vi "CRYCalc mean and abs standard.vi"(6 "Work in":u16, 7 "Step Setup VI No":i32, 8 "Statistic Run Number":i32, 11 "Data in":T1 {"Z data" items=["dB", "Lin"]; "X data" items=["dB", "Lin"]; "Y data" items=["dB", "Lin"]; "Z dB ref" format="%.1f"; "Z axis" items=["Log", "Lin"]; "X dB ref" format="%.1f"; "X axis" items=["Log", "Lin"]; "Y axis" items=["Log", "Lin"]; "Y dB ref" format="%.1f"; "Curve"."z" format="%.2f"; "Curve"."y" format="%.2f"; "Curve"."x" format="%.2f"}) -> (0 "Out F":bool, 1 "Absolute StanDev Out":T1 {"Z data" items=["dB", "Lin"]; "X data" items=["dB", "Lin"]; "Y data" items=["dB", "Lin"]; "Z dB ref" format="%.1f"; "Z axis" items=["Log", "Lin"]; "X dB ref" format="%.1f"; "X axis" items=["Log", "Lin"]; "Y axis" items=["Log", "Lin"]; "Y dB ref" format="%.1f"; "Curve"."z" format="%.2f"; "Curve"."y" format="%.2f"; "Curve"."x" format="%.2f"}, 3 "Mean Out":T1 {"Z data" items=["dB", "Lin"]; "X data" items=["dB", "Lin"]; "Y data" items=["dB", "Lin"]; "Z dB ref" format="%.1f"; "Z axis" items=["Log", "Lin"]; "X dB ref" format="%.1f"; "X axis" items=["Log", "Lin"]; "Y axis" items=["Log", "Lin"]; "Y dB ref" format="%.1f"; "Curve"."z" format="%.2f"; "Curve"."y" format="%.2f"; "Curve"."x" format="%.2f"})   [LabVIEW 2013]
uses:
  Typedef Control/CRYData Cluster Array.ctl
  Typedef Control/CRYData Cluster.ctl
  <vilib>/Analysis/5stat.llb/RMS (DBL).vi
  CRYStatistics Global.vi
  <vilib>/Analysis/NI_AALBase.lvlib
  <vilib>/Analysis/NI_AALPro.lvlib
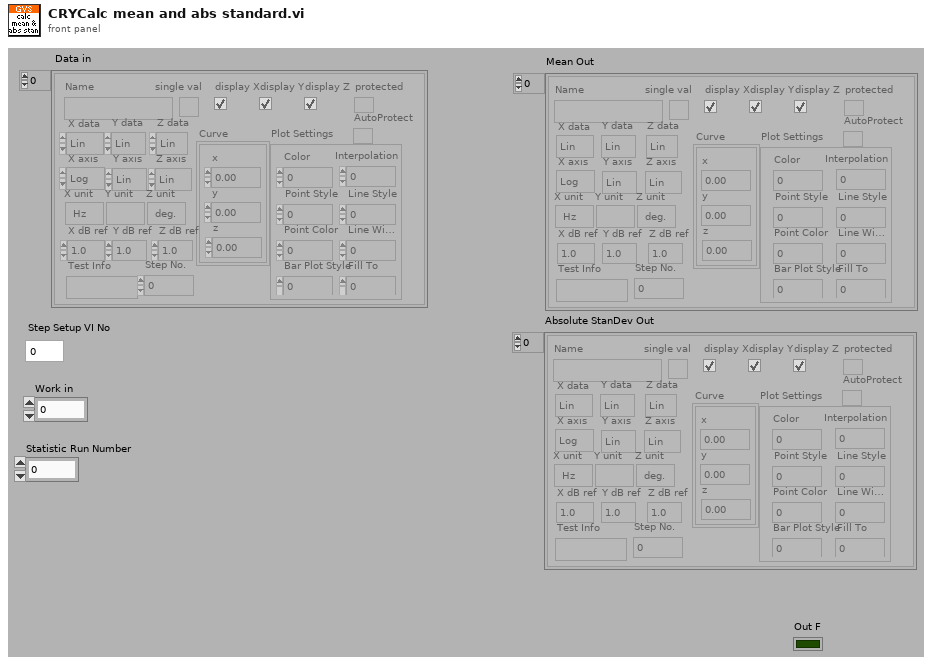
[diagram p1: front panel]
types:
  T1 = typedef "CRYData Cluster Array.ctl" = T2[]
  T2 = typedef "CRYData Cluster.ctl" = cluster{"Name":string, "Curve":cluster{"x":dbl, "y":dbl, "z":dbl}[], "X data":u16, "Y data":u16, "Z data":u16, "X axis":u16, "Y axis":u16, "Z axis":u16, "X unit":string, "Y unit":string, "Z unit":string, "X dB ref":dbl, "Y dB ref":dbl, "Z dB ref":dbl, "single val":bool, "protected":bool, "display X":bool, "display Y":bool, "display Z":bool, "Test Info":string, "Step No.":i32, "Plot Settings":cluster{"Color":u32, "Interpolation":u8, "Point Style":u8, "Line Style":u8, "Point Color":u32, "Line Width":u8, "Bar Plot Style":u8, "Fill To":i16}, "AutoProtect":bool}
  T3 = enum32{"English", "Chinese", "Korean", "Japanese", "Russian", "Chinese traditional"}
  T4 = cluster{"standard deviation":dbl, "standard deviation":dbl, "standard deviation":dbl}
  T5 = cluster{"mean":dbl, "rms value":dbl, "mean":dbl}[]
  T6 = cluster{"standard deviation":dbl, "standard deviation":dbl, "standard deviation":dbl}[]
  T7 = cluster{"x":dbl, "rms value":dbl, "rms value":dbl}
  T8 = cluster{"x":dbl, "standard deviation":dbl, "standard deviation":dbl}
  T9 = cluster{"x":dbl, "rms value":dbl, "rms value":dbl}[]
  T10 = cluster{"x":dbl, "standard deviation":dbl, "standard deviation":dbl}[]
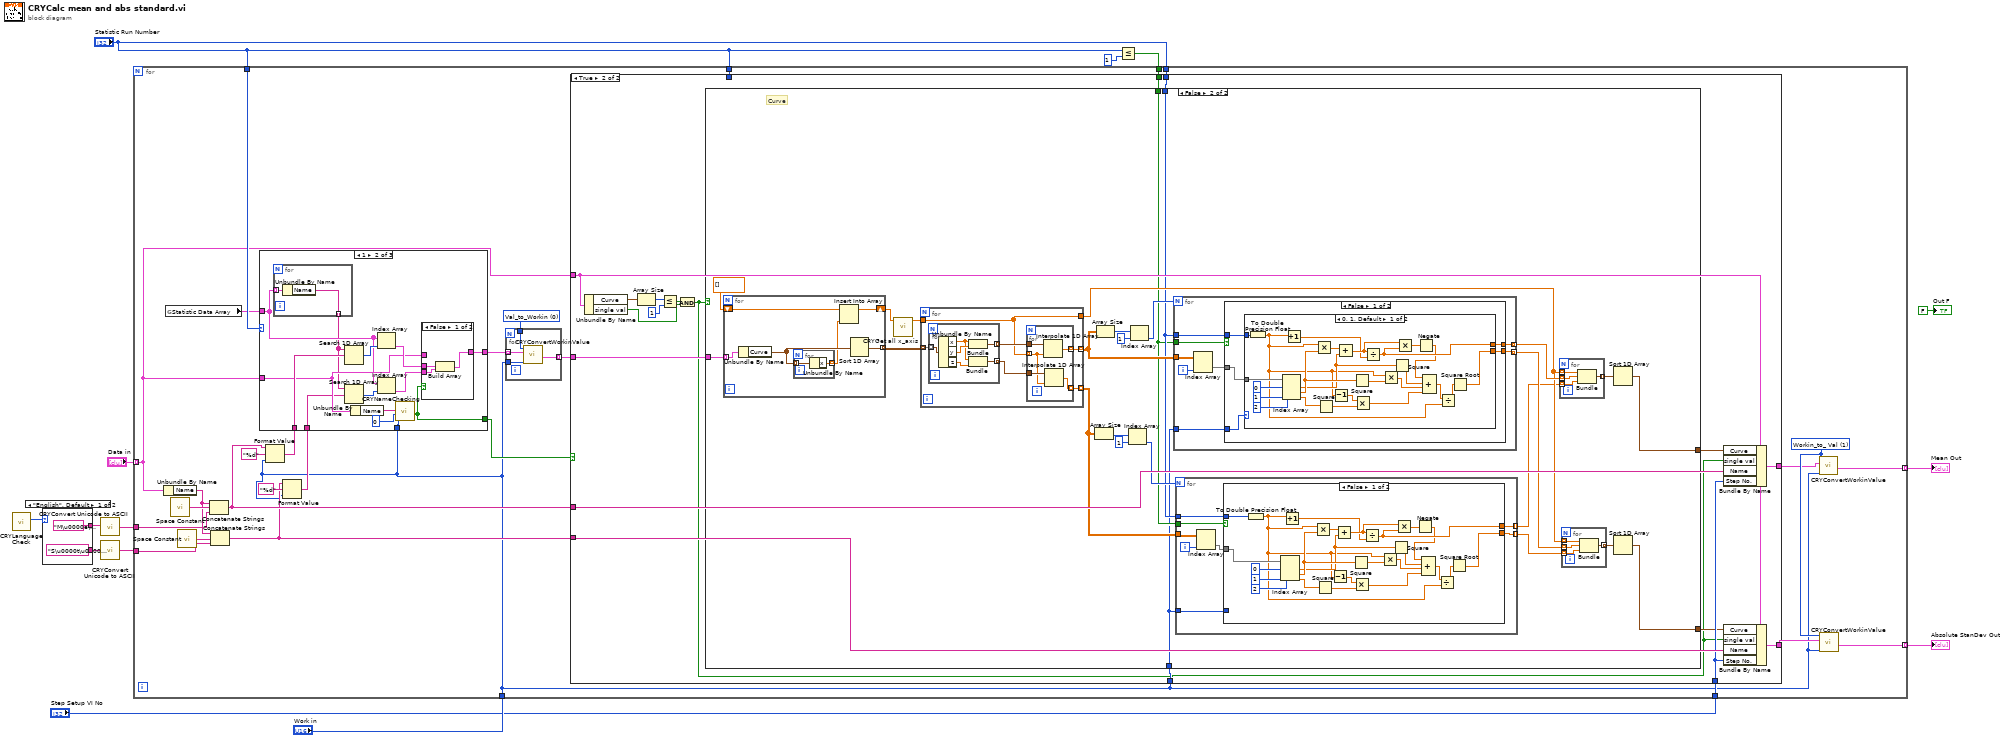
[diagram p0: block diagram]
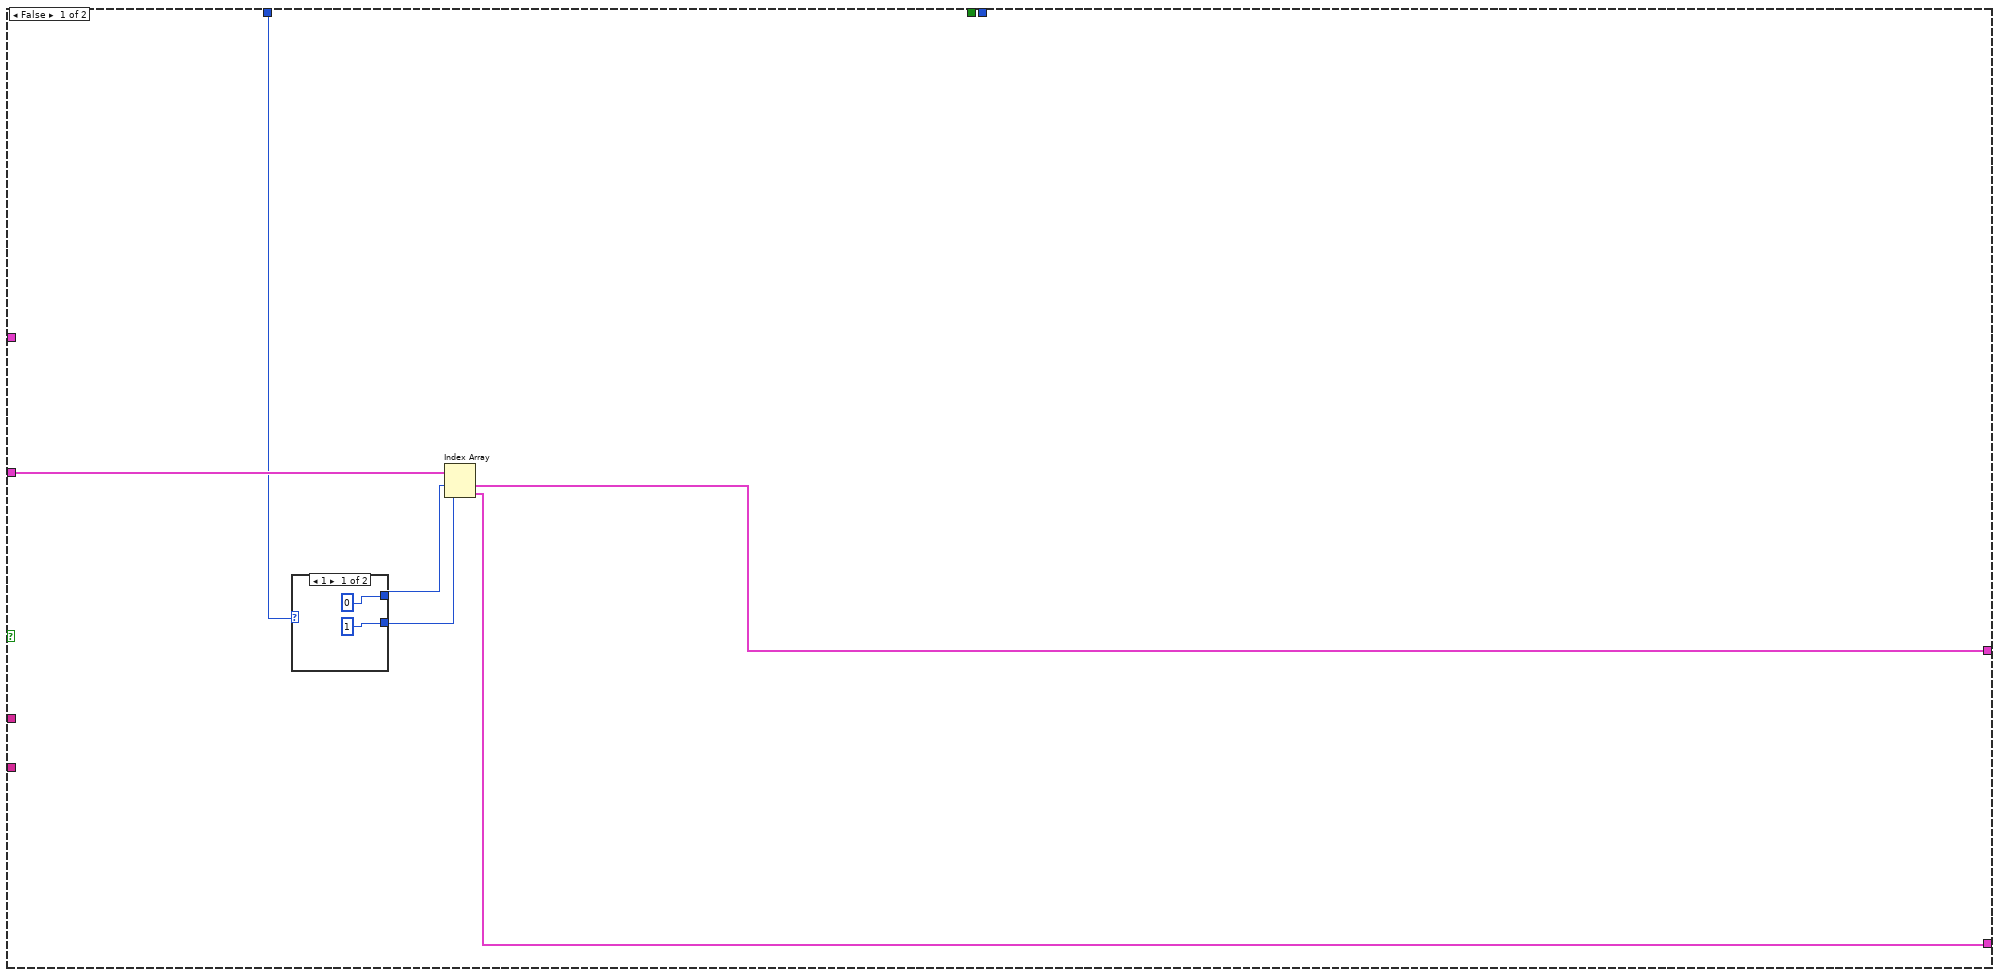
[diagram p2: hidden frame]
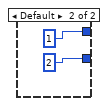
[diagram p3: hidden frame]
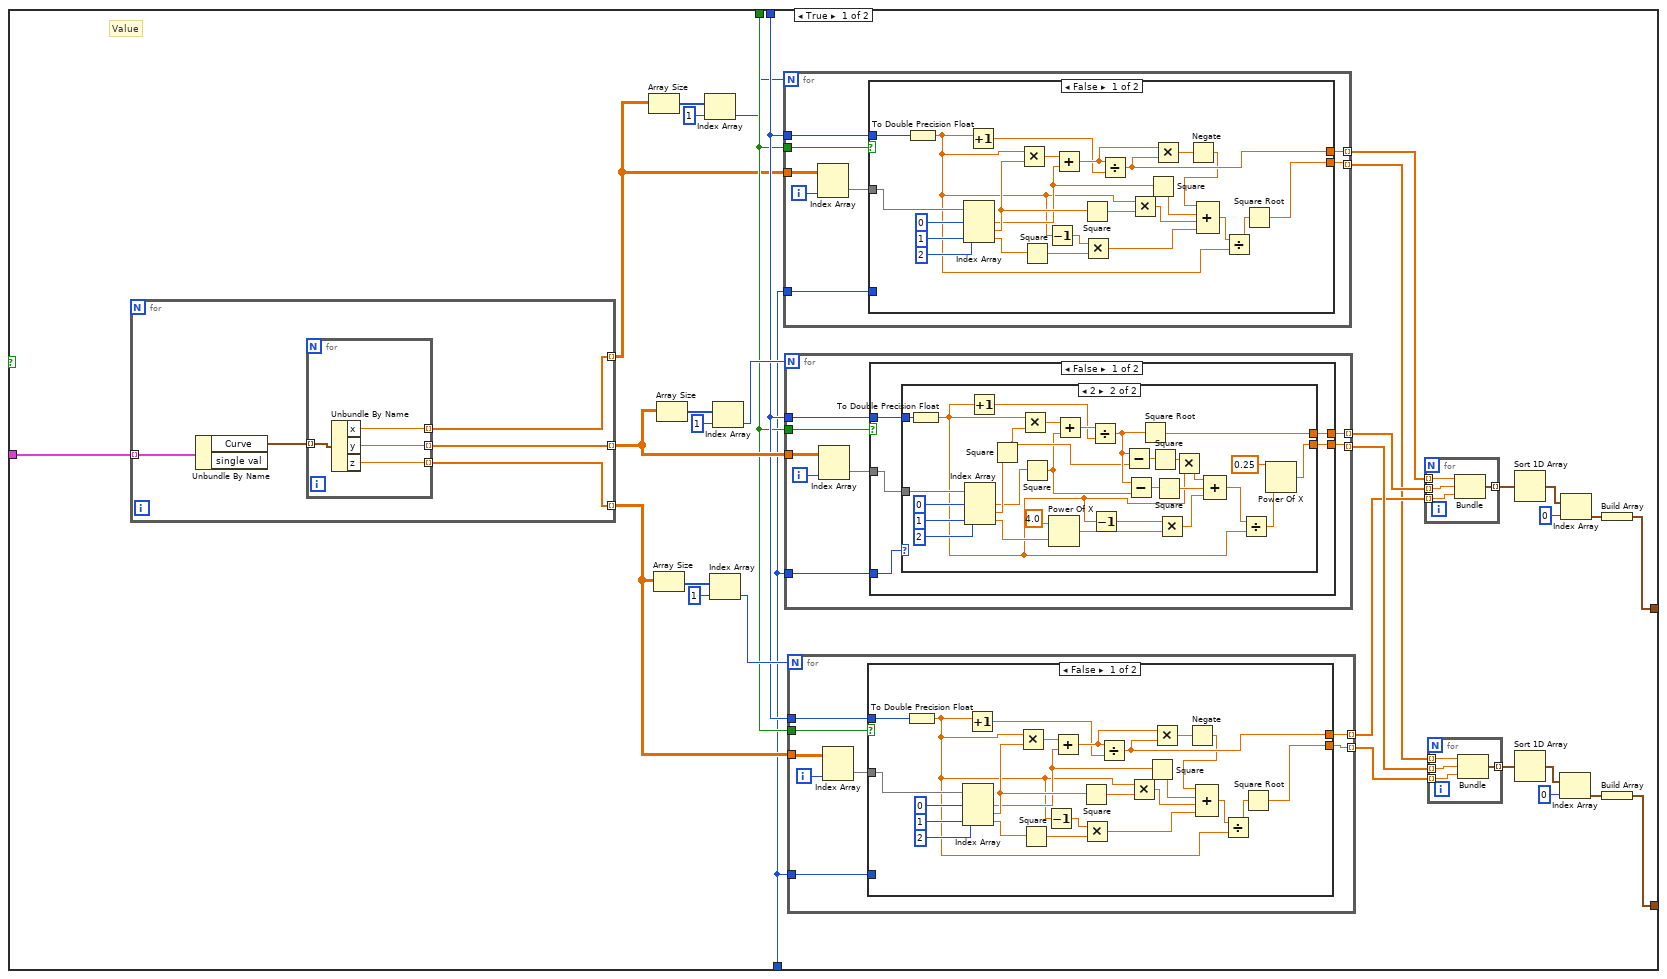
[diagram p4: hidden frame]
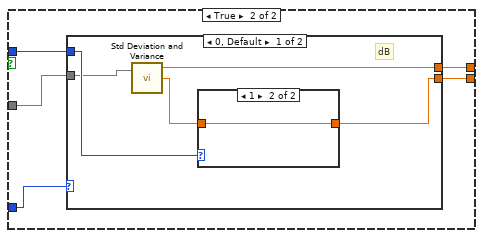
[diagram p5: hidden frame]
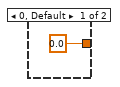
[diagram p6: hidden frame]
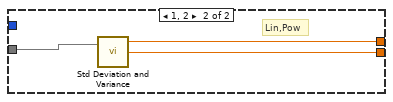
[diagram p7: hidden frame]
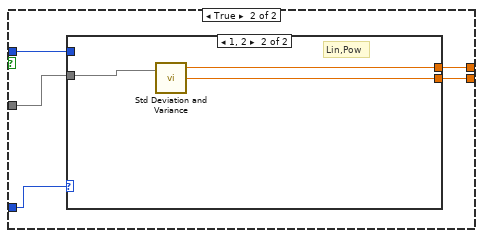
[diagram p8: hidden frame]
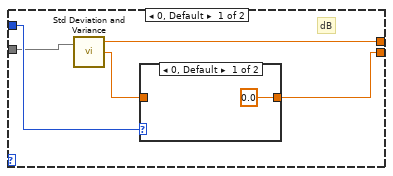
[diagram p9: hidden frame]
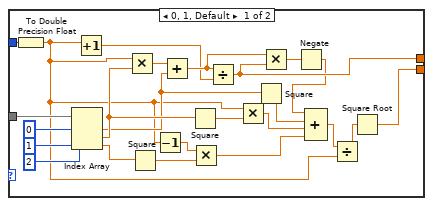
[diagram p11: hidden frame]
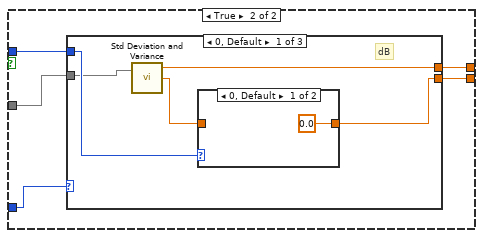
[diagram p12: hidden frame]
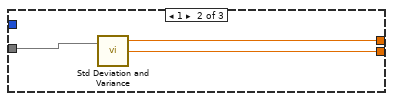
[diagram p14: hidden frame]
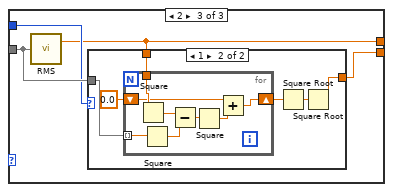
[diagram p15: hidden frame]
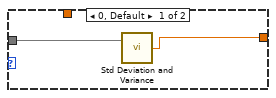
[diagram p16: hidden frame]
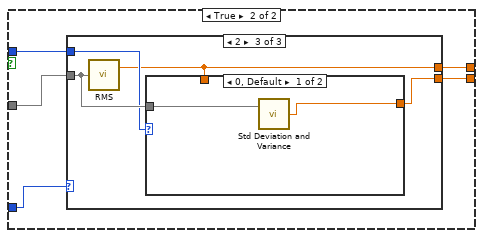
[diagram p17: hidden frame]
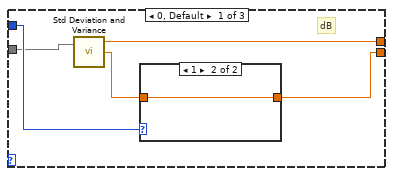
[diagram p18: hidden frame]
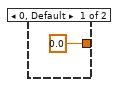
[diagram p19: hidden frame]
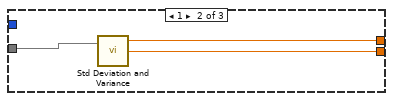
[diagram p20: hidden frame]
diagram:
  n1 = call "CRYLanguage Check.vi"() -> ("Language"=w9:T3)  [unwired: 10 in, 1 out]
  n2 = case shown="\"English\", Default" w9 {
    tunnel: ["M\u0000e\u0000a\u0000n\u0000" ("format string") "s^GW<P" ("format string")] -> w8
    tunnel: ["S\u0000t\u0000d\u0000 \u0000D\u0000e\u0000v\u0000" ("format string") "\u0007hÆQî]" ("format string")] -> w10
    frame "English", Default {
    }
    frame "Chinese" {
    }
  }
  n3 = call "CRYConvert Unicode to ASCII.vi"("Unicode"=w8) -> ("ASCII"=w7:string)  [unwired: 4 in]
  n4 = call "CRYConvert Unicode to ASCII.vi"("Unicode"=w10) -> ("ASCII"=w6:string)  [unwired: 4 in]
  n5 = Less Or Equal?(x="Statistic Run Number", y=1) -> (x <= y?=w4:bool)
  n6 = for {
    tunnel: "Data in" -> [w36] mode=indexing
    tunnel: [w27] -> w14 mode=indexing
    tunnel: w4 -> [w45]
    tunnel: "Statistic Run Number" -> [w46]
    tunnel: [w30] -> w13 mode=indexing
    tunnel: "Step Setup VI No" -> [w44]
    tunnel: "Statistic Run Number" -> [w43]
    tunnel: w7 -> [w38]
    tunnel: w6 -> [w37]
    tunnel: "Statistic Run Number" -> [w34]
    tunnel: "Work in" -> [w19]
    w31 = u16 1 items=["Val_to_Workin", "Workin_to_ Val"] ("Type")
    w33 = u16 0 items=["Val_to_Workin", "Workin_to_ Val"] ("Type")
    n7 = Unbundle By Name(w36) -> ("Name"=w40:string)
    n8 = global read "CRYStatistics Global.vi" "Statistic Data Array"() -> (w39:T1)
    n9 = call <vilib>:"Space Constant.vi"() -> ("String"=w42:string)
    n10 = call <vilib>:"Space Constant.vi"() -> ("String"=w41:string)
    n11 = Concatenate Strings(w40, w42, w38) -> (w24:string)
    n12 = Concatenate Strings(w40, w41, w37) -> (w21:string)
    n13 = Format Value(string ("")=w24, format string="%d", value (0)=w19) -> (output string=w23:string)
    n14 = Format Value(string ("")=w21, format string="%d", value (0)=w19) -> (output string=w20:string)
    n15 = case shown="1" w43 {
      tunnel: w36 -> [w550 w561 w578]
      tunnel: [w551 w564 w585] -> w29
      tunnel: w23 -> [_ w562 w586]
      tunnel: w20 -> [_ w556 w580]
      tunnel: w39 -> [_ w553 w581]
      tunnel: [TRUE ("Out Calcurated") w558 w579] -> w35
      tunnel: w19 -> [_ w554 w575]
      frame 0 {
        n16 = Build Array(w550, w550) -> (w551:T2[])
      }
      frame 1 {
        n17 = for {
          tunnel: w553 -> [w567] mode=indexing
          tunnel: [w566] -> w552 mode=indexing
          n18 = Unbundle By Name(w567) -> ("Name"=w566:string)
        }
        n19 = Search 1D Array(1D array=w552, element=w562) -> (index of element=w565:i32)  [unwired: 1 in]
        n20 = Search 1D Array(1D array=w552, element=w556) -> (index of element=w557:i32)  [unwired: 1 in]
        n21 = Unbundle By Name(w561) -> ("Name"=w560:string)
        n22 = Index Array(array=w553, index=w565) -> (element=w563:T2)
        n23 = Index Array(array=w553, index=w557) -> (element=w555:T2)
        n24 = call "CRYNameChecking.vi"("Curve Name"=w560, "Mode"=i8 0, "Work in"=w554) -> ("Out Calcurated"=w558:bool)  [unwired: 7 in]
        n25 = case shown="False" w558 {
          tunnel: [w568 w573] -> w564
          tunnel: w563 -> [w570 w572]
          tunnel: w561 -> [_ w571]
          tunnel: w555 -> [w569 _]
          frame False {
            n26 = Build Array(w570, w569) -> (w568:T2[])
          }
          frame True {
            n27 = Build Array(w571, w572) -> (w573:T2[])
          }
        }
      }
      frame Default {
        n28 = for {
          tunnel: w581 -> [w589] mode=indexing
          tunnel: [w588] -> w574 mode=indexing
          n29 = Unbundle By Name(w589) -> ("Name"=w588:string)
        }
        n30 = Unbundle By Name(w578) -> ("Name"=w577:string)
        n31 = Search 1D Array(1D array=w574, element=w586) -> (index of element=w587:i32)  [unwired: 1 in]
        n32 = Search 1D Array(1D array=w574, element=w580) -> (index of element=w583:i32)  [unwired: 1 in]
        n33 = Index Array(array=w581, index=w587) -> (element=w584:T2)
        n34 = Index Array(array=w581, index=w583) -> (element=w582:T2)
        n35 = call "CRYNameChecking.vi"("Curve Name"=w577, "Mode"=i8 0, "Work in"=w575) -> ("Out Calcurated"=w579:bool)  [unwired: 7 in]
        n36 = Build Array(w578, w584, w582) -> (w585:T2[])
      }
    }
    n37 = for {
      tunnel: w29 -> [w50] mode=indexing
      tunnel: [w49] -> w26 mode=indexing
      tunnel: w33 -> [w48]
      tunnel: w19 -> [w47]
      n38 = call "CRYConvertWorkinValue.vi"("Work in"=w47, "In"=w50, "Type"=w48) -> ("Out"=w49:T2)  [unwired: 8 in]
    }
    n39 = case shown="True" w35 {
      tunnel: [w56 w78] -> w28
      tunnel: w24 -> [_ w77]
      tunnel: w21 -> [_ w76]
      tunnel: [w55 w75] -> w32
      tunnel: w46 -> [_ w74]
      tunnel: w45 -> [_ w69]
      tunnel: w26 -> [w54 w73]
      tunnel: w44 -> [_ w72]
      tunnel: w36 -> [_ w62]
      tunnel: w34 -> [w53 _]
      tunnel: w19 -> [_ w68]
      frame False {
        n40 = case shown="1" w53 {
          tunnel: [0 1] -> w52
          tunnel: [1 2] -> w51
          frame 1 {
          }
          frame Default {
          }
        }
        n41 = Index Array(array=w54, index #1=w52, index #2=w51) -> (element #1=w56:T2, element #2=w55:T2)
      }
      frame True {
        n42 = Unbundle By Name(w62) -> ("Curve"=w67:cluster{"x":dbl, "y":dbl, "z":dbl}[], "single val"=w63:bool)
        n43 = Array Size(array=w67) -> (size(s)=w66:i32)
        n44 = Less Or Equal?(x=w66, y=1) -> (x <= y?=w64:bool)
        n45 = And(x=w64, y=w63) -> (x .and. y?=w61:bool)
        n46 = case shown="False" w61 {
          tunnel: w74 -> [w87 w331]
          tunnel: w73 -> [w92 w327]
          tunnel: [w95 w326] -> w71
          tunnel: [w93 w325] -> w70
          tunnel: w69 -> [w86 w324]
          tunnel: w68 -> [w85 w323]
          frame True {
            # "Value"
            n47 = for {
              tunnel: [w315] -> w110 mode=indexing
              tunnel: [w314] -> w99 mode=indexing
              tunnel: w92 -> [w318] mode=indexing
              tunnel: [w316] -> w81 mode=indexing
              n48 = Unbundle By Name(w318) -> ("Curve"=w317:cluster{"x":dbl, "y":dbl, "z":dbl}[])  [unwired: 1 out]
              n49 = for {
                tunnel: w317 -> [w322] mode=indexing
                tunnel: [w321] -> w316 mode=indexing
                tunnel: [w320] -> w315 mode=indexing
                tunnel: [w319] -> w314 mode=indexing
                n50 = Unbundle By Name(w322) -> ("x"=w321:dbl, "y"=w320:dbl, "z"=w319:dbl)
              }
            }
            n51 = Array Size(array=w81) -> (size(s)=w83:i32[])
            n52 = Array Size(array=w99) -> (size(s)=w103:i32[])
            n53 = Array Size(array=w110) -> (size(s)=w109:i32[])
            n54 = Index Array(array=w83, index=1) -> (element=w82:i32)
            n55 = Index Array(array=w103, index=1) -> (element=w100:i32)
            n56 = Index Array(array=w109, index=1) -> (element=w108:i32)
            n57 = for {
              N: w82 -> [_]
              tunnel: w81 -> [w118]
              tunnel: [w115] -> w79 mode=indexing
              tunnel: w86 -> [w114]
              tunnel: w87 -> [w113]
              tunnel: [w112] -> w80 mode=indexing
              tunnel: w85 -> [w111]
              i -> [w117]
              n58 = Index Array(array=w118, index (col)=w117) -> (element=w116:dbl[])  [unwired: 1 in]
              n59 = case shown="False" w114 {
                tunnel: w116 -> [w142 w147]
                tunnel: [w141 w146] -> w115
                tunnel: w113 -> [w139 w143]
                tunnel: [w140 w145] -> w112
                tunnel: w111 -> [_ w144]
                frame False {
                  n60 = To Double Precision Float(number=w139) -> (double precision float=w119:dbl)
                  n61 = Index Array(array=w142, index #1=0 ("index"), index #2=1 ("index"), index #3=2 ("index")) -> (element #1=w129:dbl, element #2=w131:dbl, element #3=w134:dbl)
                  n62 = Increment(x=w119) -> (x+1=w120:dbl)
                  n63 = Multiply(x=w119, y=w131) -> (x*y=w135:dbl)
                  n64 = Square(x=w134) -> (x^2=w132:dbl)
                  n65 = Decrement(x=w119) -> (x-1=w133:dbl)
                  n66 = Add(x=w135, y=w129) -> (x+y=w125:dbl)
                  n67 = Square(x=w131) -> (x^2=w130:dbl)
                  n68 = Multiply(x=w133, y=w132) -> (x*y=w126:dbl)
                  n69 = Divide(x=w125, y=w120) -> (x/y=w141:dbl)
                  n70 = Multiply(x=w119, y=w130) -> (x*y=w127:dbl)
                  n71 = Square(x=w129) -> (x^2=w128:dbl)
                  n72 = Multiply(x=w125, y=w141) -> (x*y=w124:dbl)
                  n73 = Negate(x=w124) -> (-x=w123:dbl)
                  n74 = Compound Arithmetic op=ADD(w123, w128, w127, w126) -> (w122:dbl)
                  n75 = Divide(x=w122, y=w119) -> (x/y=w121:dbl)
                  n76 = Square Root(x=w121) -> (sqrt(x)=w140:dbl)
                }
                frame True {
                  n77 = case shown="0, Default" w144 {
                    tunnel: w147 -> [w149 w157]
                    tunnel: [w152 w156] -> w146
                    tunnel: [w150 w155] -> w145
                    tunnel: w143 -> [w151 _]
                    frame 0, Default {
                      # "dB"
                      n78 = call <vilib>:"Std Deviation and Variance.vi"("X"=w149) -> ("mean"=w152:dbl, "standard deviation"=w148:dbl)  [unwired: 1 in, 1 out]
                      n79 = case shown="1" w151 {
                        tunnel: [0.0 w154] -> w150
                        tunnel: w148 -> [_ w154]
                        frame 0, Default {
                        }
                        frame 1 {
                        }
                      }
                    }
                    frame 1, 2 {
                      # "Lin,Pow"
                      n80 = call <vilib>:"Std Deviation and Variance.vi"("X"=w157) -> ("mean"=w156:dbl, "standard deviation"=w155:dbl)  [unwired: 1 in, 1 out]
                    }
                  }
                }
              }
            }
            n81 = for {
              N: w108 -> [_]
              tunnel: w110 -> [w220]
              tunnel: [w217] -> w106 mode=indexing
              tunnel: w86 -> [w216]
              tunnel: w87 -> [w215]
              tunnel: [w214] -> w101 mode=indexing
              tunnel: w85 -> [w213]
              i -> [w219]
              n82 = Index Array(array=w220, index (col)=w219) -> (element=w218:dbl[])  [unwired: 1 in]
              n83 = case shown="False" w216 {
                tunnel: w218 -> [w225 w283]
                tunnel: [w224 w282] -> w217
                tunnel: w215 -> [w222 w279]
                tunnel: [w223 w281] -> w214
                tunnel: w213 -> [w221 w280]
                frame False {
                  n84 = case shown="2" w221 {
                    tunnel: w225 -> [w249 w278]
                    tunnel: [w234 w269] -> w224
                    tunnel: [w230 w261] -> w223
                    tunnel: w222 -> [w228 w264]
                    frame 0, 1, Default {
                      n85 = To Double Precision Float(number=w228) -> (double precision float=w226:dbl)
                      n86 = Index Array(array=w249, index #1=0 ("index"), index #2=1 ("index"), index #3=2 ("index")) -> (element #1=w239:dbl, element #2=w241:dbl, element #3=w244:dbl)
                      n87 = Increment(x=w226) -> (x+1=w227:dbl)
                      n88 = Multiply(x=w226, y=w241) -> (x*y=w245:dbl)
                      n89 = Square(x=w244) -> (x^2=w242:dbl)
                      n90 = Decrement(x=w226) -> (x-1=w243:dbl)
                      n91 = Add(x=w245, y=w239) -> (x+y=w235:dbl)
                      n92 = Square(x=w241) -> (x^2=w240:dbl)
                      n93 = Multiply(x=w243, y=w242) -> (x*y=w236:dbl)
                      n94 = Divide(x=w235, y=w227) -> (x/y=w234:dbl)
                      n95 = Multiply(x=w226, y=w240) -> (x*y=w237:dbl)
                      n96 = Square(x=w239) -> (x^2=w238:dbl)
                      n97 = Multiply(x=w235, y=w234) -> (x*y=w233:dbl)
                      n98 = Negate(x=w233) -> (-x=w232:dbl)
                      n99 = Compound Arithmetic op=ADD(w232, w238, w237, w236) -> (w231:dbl)
                      n100 = Divide(x=w231, y=w226) -> (x/y=w229:dbl)
                      n101 = Square Root(x=w229) -> (sqrt(x)=w230:dbl)
                    }
                    frame 2 {
                      n102 = To Double Precision Float(number=w264) -> (double precision float=w251:dbl)
                      n103 = Index Array(array=w278, index #1=0 ("index"), index #2=1 ("index"), index #3=2 ("index")) -> (element #1=w272:dbl, element #2=w273:dbl, element #3=w268:dbl)
                      n104 = Increment(x=w251) -> (x+1=w254:dbl)
                      n105 = Square(x=w273) -> (x^2=w257:dbl)
                      n106 = Multiply(x=w251, y=w257) -> (x*y=w274:dbl)
                      n107 = Square(x=w272) -> (x^2=w256:dbl)
                      n108 = Power Of X(1:w268, 2:4.0 ("y")) -> (0:w266:dbl)
                      n109 = Add(x=w274, y=w256) -> (x+y=w271:dbl)
                      n110 = Divide(x=w271, y=w254) -> (x/y=w258:dbl)
                      n111 = Decrement(x=w251) -> (x-1=w250:dbl)
                      n112 = Subtract(x=w258, y=w257) -> (x-y=w259:dbl)
                      n113 = Subtract(x=w258, y=w256) -> (x-y=w253:dbl)
                      n114 = Square Root(x=w258) -> (sqrt(x)=w269:dbl)
                      n115 = Square(x=w259) -> (x^2=w260:dbl)
                      n116 = Square(x=w253) -> (x^2=w252:dbl)
                      n117 = Multiply(x=w250, y=w266) -> (x*y=w265:dbl)
                      n118 = Multiply(x=w260, y=w251) -> (x*y=w255:dbl)
                      n119 = Compound Arithmetic op=ADD(w255, w252, w265) -> (w270:dbl)
                      n120 = Divide(x=w270, y=w251) -> (x/y=w263:dbl)
                      n121 = Power Of X(1:w263, 2:0.25 ("y")) -> (0:w261:dbl)
                    }
                  }
                }
                frame True {
                  n122 = case shown="0, Default" w280 {
                    tunnel: w283 -> [w285 w293 w296]
                    tunnel: [w288 w292 w294] -> w282
                    tunnel: [w286 w291 w297] -> w281
                    tunnel: w279 -> [w287 _ w295]
                    frame 0, Default {
                      # "dB"
                      n123 = call <vilib>:"Std Deviation and Variance.vi"("X"=w285) -> ("mean"=w288:dbl, "standard deviation"=w284:dbl)  [unwired: 1 in, 1 out]
                      n124 = case shown="0, Default" w287 {
                        tunnel: [0.0 w290] -> w286
                        tunnel: w284 -> [_ w290]
                        frame 0, Default {
                        }
                        frame 1 {
                        }
                      }
                    }
                    frame 1 {
                      n125 = call <vilib>:"Std Deviation and Variance.vi"("X"=w293) -> ("mean"=w292:dbl, "standard deviation"=w291:dbl)  [unwired: 1 in, 1 out]
                    }
                    frame 2 {
                      n126 = call-poly <vilib>:"RMS.vi"("X"=w296) -> ("rms value"=w294:dbl)  [unwired: 1 out]
                      n127 = case shown="1" w295 {
                        tunnel: [w298 w300] -> w297
                        tunnel: w296 -> [w299 w304]
                        tunnel: w294 -> [_ w303]
                        frame 0, Default {
                          n128 = call <vilib>:"Std Deviation and Variance.vi"("X"=w299) -> ("standard deviation"=w298:dbl)  [unwired: 1 in, 2 out]
                        }
                        frame 1 {
                          n129 = for {
                            tunnel: w304 -> [w312] mode=indexing
                            tunnel: w303 -> [w313]
                            shift-right: [w308] -> w302
                            shift-left: 0.0 -> [w307]
                            n130 = Square(x=w313) -> (x^2=w311:dbl)
                            n131 = Square(x=w312) -> (x^2=w310:dbl)
                            n132 = Subtract(x=w311, y=w310) -> (x-y=w309:dbl)
                            n133 = Square(x=w309) -> (x^2=w306:dbl)
                            n134 = Add(x=w307, y=w306) -> (x+y=w308:dbl)
                          }
                          n135 = Square Root(x=w302) -> (sqrt(x)=w301:dbl)
                          n136 = Square Root(x=w301) -> (sqrt(x)=w300:dbl)
                        }
                      }
                    }
                  }
                }
              }
            }
            n137 = for {
              N: w100 -> [_]
              tunnel: w99 -> [w165]
              tunnel: [w160] -> w98 mode=indexing
              tunnel: w86 -> [w162]
              tunnel: w87 -> [w163]
              tunnel: [w159] -> w97 mode=indexing
              tunnel: w85 -> [w161]
              i -> [w164]
              n138 = Index Array(array=w165, index (col)=w164) -> (element=w158:dbl[])  [unwired: 1 in]
              n139 = case shown="False" w162 {
                tunnel: w158 -> [w189 w194]
                tunnel: [w188 w193] -> w160
                tunnel: w163 -> [w186 w190]
                tunnel: [w187 w192] -> w159
                tunnel: w161 -> [_ w191]
                frame False {
                  n140 = To Double Precision Float(number=w186) -> (double precision float=w166:dbl)
                  n141 = Index Array(array=w189, index #1=0 ("index"), index #2=1 ("index"), index #3=2 ("index")) -> (element #1=w176:dbl, element #2=w178:dbl, element #3=w181:dbl)
                  n142 = Increment(x=w166) -> (x+1=w167:dbl)
                  n143 = Multiply(x=w166, y=w178) -> (x*y=w182:dbl)
                  n144 = Square(x=w181) -> (x^2=w179:dbl)
                  n145 = Decrement(x=w166) -> (x-1=w180:dbl)
                  n146 = Add(x=w182, y=w176) -> (x+y=w172:dbl)
                  n147 = Square(x=w178) -> (x^2=w177:dbl)
                  n148 = Multiply(x=w180, y=w179) -> (x*y=w173:dbl)
                  n149 = Divide(x=w172, y=w167) -> (x/y=w188:dbl)
                  n150 = Multiply(x=w166, y=w177) -> (x*y=w174:dbl)
                  n151 = Square(x=w176) -> (x^2=w175:dbl)
                  n152 = Multiply(x=w172, y=w188) -> (x*y=w171:dbl)
                  n153 = Negate(x=w171) -> (-x=w170:dbl)
                  n154 = Compound Arithmetic op=ADD(w170, w175, w174, w173) -> (w169:dbl)
                  n155 = Divide(x=w169, y=w166) -> (x/y=w168:dbl)
                  n156 = Square Root(x=w168) -> (sqrt(x)=w187:dbl)
                }
                frame True {
                  n157 = case shown="1, 2" w191 {
                    tunnel: w194 -> [w196 w204]
                    tunnel: [w199 w203] -> w193
                    tunnel: [w197 w202] -> w192
                    tunnel: w190 -> [w198 _]
                    frame 0, Default {
                      # "dB"
                      n158 = call <vilib>:"Std Deviation and Variance.vi"("X"=w196) -> ("mean"=w199:dbl, "standard deviation"=w195:dbl)  [unwired: 1 in, 1 out]
                      n159 = case shown="0, Default" w198 {
                        tunnel: [0.0 w201] -> w197
                        tunnel: w195 -> [_ w201]
                        frame 0, Default {
                        }
                        frame 1 {
                        }
                      }
                    }
                    frame 1, 2 {
                      # "Lin,Pow"
                      n160 = call <vilib>:"Std Deviation and Variance.vi"("X"=w204) -> ("mean"=w203:dbl, "standard deviation"=w202:dbl)  [unwired: 1 in, 1 out]
                    }
                  }
                }
              }
            }
            n161 = for {
              tunnel: w106 -> [w211] mode=indexing
              tunnel: [w212] -> w105 mode=indexing
              tunnel: w79 -> [w210] mode=indexing
              tunnel: w98 -> [w209] mode=indexing
              n162 = Bundle("mean"=w210, "rms value"=w211, "mean"=w209) -> (w212:cluster{"mean":dbl, "rms value":dbl, "mean":dbl})  [unwired: 1 out]
            }
            n163 = for {
              tunnel: w101 -> [w207] mode=indexing
              tunnel: [w208] -> w102 mode=indexing
              tunnel: w80 -> [w206] mode=indexing
              tunnel: w97 -> [w205] mode=indexing
              n164 = Bundle("standard deviation"=w206, "standard deviation"=w207, "standard deviation"=w205) -> (w208:T4)  [unwired: 1 out]
            }
            n165 = Sort 1D Array(array=w105) -> (sorted array=w96:T5)
            n166 = Sort 1D Array(array=w102) -> (sorted array=w94:T6)
            n167 = Index Array(array=w94, index=0) -> (element=w88:T4)
            n168 = Index Array(array=w96, index=0) -> (element=w90:cluster{"mean":dbl, "rms value":dbl, "mean":dbl})
            n169 = Build Array(w90) -> (w95:T5)
            n170 = Build Array(w88) -> (w93:T6)
          }
          frame False {
            # "Curve"
            n171 = for {
              tunnel: [w524] -> w345 mode=indexing
              tunnel: w327 -> [w525] mode=indexing
              shift-right: [w527] -> w338
              shift-left: dbl[] [] ("x_Array") -> [w526]
              n172 = Unbundle By Name(w525) -> ("Curve"=w529:cluster{"x":dbl, "y":dbl, "z":dbl}[])
              n173 = for {
                tunnel: w529 -> [w530] mode=indexing
                tunnel: [w531] -> w528 mode=indexing
                n174 = Unbundle By Name(w530) -> ("x"=w531:dbl)
              }
              n175 = Insert Into Array(array=w526, new element=w528) -> (w527:dbl[])  [unwired: 1 in]
              n176 = Sort 1D Array(array=w529) -> (sorted array=w524:cluster{"x":dbl, "y":dbl, "z":dbl}[])
            }
            n177 = call "CRYGet all x_axis.vi"("x_Array in"=w338) -> ("X_axis out"=w344:dbl[])  [unwired: 1 in, 9 out]
            n178 = for {
              tunnel: w345 -> [w533] mode=indexing
              tunnel: [w537] -> w347 mode=indexing
              tunnel: w344 -> [w532]
              tunnel: [w532] -> w334
              tunnel: [w534] -> w330 mode=indexing
              n179 = for {
                tunnel: [w542] -> w536 mode=indexing
                tunnel: w533 -> [w541] mode=indexing
                tunnel: [w538] -> w535 mode=indexing
                n180 = Unbundle By Name(w541) -> ("x"=w539:dbl, "y"=w543:dbl, "z"=w540:dbl)
                n181 = Bundle("x"=w539, "z"=w540) -> (w538:cluster{"x":dbl, "z":dbl})  [unwired: 1 out]
                n182 = Bundle("x"=w539, "y"=w543) -> (w542:cluster{"x":dbl, "y":dbl})  [unwired: 1 out]
              }
              n183 = for {
                tunnel: [w548] -> w537 mode=indexing
                tunnel: w536 -> [w547]
                tunnel: w532 -> [w545] mode=indexing
                tunnel: w535 -> [w546]
                tunnel: [w544] -> w534 mode=indexing
                n184 = Interpolate 1D Array(1:w545, 2:w547) -> (0:w548:dbl)
                n185 = Interpolate 1D Array(1:w545, 2:w546) -> (0:w544:dbl)
              }
            }
            n186 = Array Size(array=w330) -> (size(s)=w336:i32[])
            n187 = Array Size(array=w347) -> (size(s)=w343:i32[])
            n188 = Index Array(array=w336, index=1) -> (element=w332:i32)
            n189 = Index Array(array=w343, index=1) -> (element=w342:i32)
            n190 = for {
              N: w342 -> [_]
              tunnel: w347 -> [w430]
              tunnel: [w427] -> w340 mode=indexing
              tunnel: w324 -> [w426]
              tunnel: w331 -> [w425]
              tunnel: [w424] -> w333 mode=indexing
              tunnel: w323 -> [w423]
              i -> [w429]
              n191 = Index Array(array=w430, index (col)=w429) -> (element=w428:dbl[])  [unwired: 1 in]
              n192 = case shown="False" w426 {
                tunnel: w428 -> [w435 w493]
                tunnel: [w434 w492] -> w427
                tunnel: w425 -> [w432 w489]
                tunnel: [w433 w491] -> w424
                tunnel: w423 -> [w431 w490]
                frame False {
                  n193 = case shown="0, 1, Default" w431 {
                    tunnel: w435 -> [w459 w488]
                    tunnel: [w444 w479] -> w434
                    tunnel: [w440 w471] -> w433
                    tunnel: w432 -> [w438 w474]
                    frame 0, 1, Default {
                      n194 = To Double Precision Float(number=w438) -> (double precision float=w436:dbl)
                      n195 = Index Array(array=w459, index #1=0 ("index"), index #2=1 ("index"), index #3=2 ("index")) -> (element #1=w449:dbl, element #2=w451:dbl, element #3=w454:dbl)
                      n196 = Increment(x=w436) -> (x+1=w437:dbl)
                      n197 = Multiply(x=w436, y=w451) -> (x*y=w455:dbl)
                      n198 = Square(x=w454) -> (x^2=w452:dbl)
                      n199 = Decrement(x=w436) -> (x-1=w453:dbl)
                      n200 = Add(x=w455, y=w449) -> (x+y=w445:dbl)
                      n201 = Square(x=w451) -> (x^2=w450:dbl)
                      n202 = Multiply(x=w453, y=w452) -> (x*y=w446:dbl)
                      n203 = Divide(x=w445, y=w437) -> (x/y=w444:dbl)
                      n204 = Multiply(x=w436, y=w450) -> (x*y=w447:dbl)
                      n205 = Square(x=w449) -> (x^2=w448:dbl)
                      n206 = Multiply(x=w445, y=w444) -> (x*y=w443:dbl)
                      n207 = Negate(x=w443) -> (-x=w442:dbl)
                      n208 = Compound Arithmetic op=ADD(w442, w448, w447, w446) -> (w441:dbl)
                      n209 = Divide(x=w441, y=w436) -> (x/y=w439:dbl)
                      n210 = Square Root(x=w439) -> (sqrt(x)=w440:dbl)
                    }
                    frame 2 {
                      n211 = To Double Precision Float(number=w474) -> (double precision float=w461:dbl)
                      n212 = Index Array(array=w488, index #1=0 ("index"), index #2=1 ("index"), index #3=2 ("index")) -> (element #1=w482:dbl, element #2=w483:dbl, element #3=w478:dbl)
                      n213 = Increment(x=w461) -> (x+1=w464:dbl)
                      n214 = Square(x=w483) -> (x^2=w467:dbl)
                      n215 = Multiply(x=w461, y=w467) -> (x*y=w484:dbl)
                      n216 = Square(x=w482) -> (x^2=w466:dbl)
                      n217 = Power Of X(1:w478, 2:4.0 ("y")) -> (0:w476:dbl)
                      n218 = Add(x=w484, y=w466) -> (x+y=w481:dbl)
                      n219 = Divide(x=w481, y=w464) -> (x/y=w468:dbl)
                      n220 = Decrement(x=w461) -> (x-1=w460:dbl)
                      n221 = Subtract(x=w468, y=w467) -> (x-y=w469:dbl)
                      n222 = Subtract(x=w468, y=w466) -> (x-y=w463:dbl)
                      n223 = Square Root(x=w468) -> (sqrt(x)=w479:dbl)
                      n224 = Square(x=w469) -> (x^2=w470:dbl)
                      n225 = Square(x=w463) -> (x^2=w462:dbl)
                      n226 = Multiply(x=w460, y=w476) -> (x*y=w475:dbl)
                      n227 = Multiply(x=w470, y=w461) -> (x*y=w465:dbl)
                      n228 = Compound Arithmetic op=ADD(w465, w462, w475) -> (w480:dbl)
                      n229 = Divide(x=w480, y=w461) -> (x/y=w473:dbl)
                      n230 = Power Of X(1:w473, 2:0.25 ("y")) -> (0:w471:dbl)
                    }
                  }
                }
                frame True {
                  n231 = case shown="2" w490 {
                    tunnel: w493 -> [w495 w503 w506]
                    tunnel: [w498 w502 w504] -> w492
                    tunnel: [w496 w501 w507] -> w491
                    tunnel: w489 -> [w497 _ w505]
                    frame 0, Default {
                      # "dB"
                      n232 = call <vilib>:"Std Deviation and Variance.vi"("X"=w495) -> ("mean"=w498:dbl, "standard deviation"=w494:dbl)  [unwired: 1 in, 1 out]
                      n233 = case shown="1" w497 {
                        tunnel: [0.0 w500] -> w496
                        tunnel: w494 -> [_ w500]
                        frame 0, Default {
                        }
                        frame 1 {
                        }
                      }
                    }
                    frame 1 {
                      n234 = call <vilib>:"Std Deviation and Variance.vi"("X"=w503) -> ("mean"=w502:dbl, "standard deviation"=w501:dbl)  [unwired: 1 in, 1 out]
                    }
                    frame 2 {
                      n235 = call-poly <vilib>:"RMS.vi"("X"=w506) -> ("rms value"=w504:dbl)  [unwired: 1 out]
                      n236 = case shown="0, Default" w505 {
                        tunnel: [w508 w510] -> w507
                        tunnel: w506 -> [w509 w514]
                        tunnel: w504 -> [_ w513]
                        frame 0, Default {
                          n237 = call <vilib>:"Std Deviation and Variance.vi"("X"=w509) -> ("standard deviation"=w508:dbl)  [unwired: 1 in, 2 out]
                        }
                        frame 1 {
                          n238 = for {
                            tunnel: w514 -> [w522] mode=indexing
                            tunnel: w513 -> [w523]
                            shift-right: [w518] -> w512
                            shift-left: 0.0 -> [w517]
                            n239 = Square(x=w523) -> (x^2=w521:dbl)
                            n240 = Square(x=w522) -> (x^2=w520:dbl)
                            n241 = Subtract(x=w521, y=w520) -> (x-y=w519:dbl)
                            n242 = Square(x=w519) -> (x^2=w516:dbl)
                            n243 = Add(x=w517, y=w516) -> (x+y=w518:dbl)
                          }
                          n244 = Square Root(x=w512) -> (sqrt(x)=w511:dbl)
                          n245 = Square Root(x=w511) -> (sqrt(x)=w510:dbl)
                        }
                      }
                    }
                  }
                }
              }
            }
            n246 = for {
              N: w332 -> [_]
              tunnel: w330 -> [w355]
              tunnel: [w350] -> w329 mode=indexing
              tunnel: w324 -> [w352]
              tunnel: w331 -> [w353]
              tunnel: [w349] -> w328 mode=indexing
              tunnel: w323 -> [w351]
              i -> [w354]
              n247 = Index Array(array=w355, index (col)=w354) -> (element=w348:dbl[])  [unwired: 1 in]
              n248 = case shown="False" w352 {
                tunnel: w348 -> [w379 w384]
                tunnel: [w378 w383] -> w350
                tunnel: w353 -> [w376 w380]
                tunnel: [w377 w382] -> w349
                tunnel: w351 -> [_ w381]
                frame False {
                  n249 = To Double Precision Float(number=w376) -> (double precision float=w356:dbl)
                  n250 = Index Array(array=w379, index #1=0 ("index"), index #2=1 ("index"), index #3=2 ("index")) -> (element #1=w366:dbl, element #2=w368:dbl, element #3=w371:dbl)
                  n251 = Increment(x=w356) -> (x+1=w357:dbl)
                  n252 = Multiply(x=w356, y=w368) -> (x*y=w372:dbl)
                  n253 = Square(x=w371) -> (x^2=w369:dbl)
                  n254 = Decrement(x=w356) -> (x-1=w370:dbl)
                  n255 = Add(x=w372, y=w366) -> (x+y=w362:dbl)
                  n256 = Square(x=w368) -> (x^2=w367:dbl)
                  n257 = Multiply(x=w370, y=w369) -> (x*y=w363:dbl)
                  n258 = Divide(x=w362, y=w357) -> (x/y=w378:dbl)
                  n259 = Multiply(x=w356, y=w367) -> (x*y=w364:dbl)
                  n260 = Square(x=w366) -> (x^2=w365:dbl)
                  n261 = Multiply(x=w362, y=w378) -> (x*y=w361:dbl)
                  n262 = Negate(x=w361) -> (-x=w360:dbl)
                  n263 = Compound Arithmetic op=ADD(w360, w365, w364, w363) -> (w359:dbl)
                  n264 = Divide(x=w359, y=w356) -> (x/y=w358:dbl)
                  n265 = Square Root(x=w358) -> (sqrt(x)=w377:dbl)
                }
                frame True {
                  n266 = case shown="2" w381 {
                    tunnel: w384 -> [w386 w394 w397]
                    tunnel: [w389 w393 w395] -> w383
                    tunnel: [w387 w392 w398] -> w382
                    tunnel: w380 -> [w388 _ w396]
                    frame 0, Default {
                      # "dB"
                      n267 = call <vilib>:"Std Deviation and Variance.vi"("X"=w386) -> ("mean"=w389:dbl, "standard deviation"=w385:dbl)  [unwired: 1 in, 1 out]
                      n268 = case shown="1" w388 {
                        tunnel: [0.0 w391] -> w387
                        tunnel: w385 -> [_ w391]
                        frame 0, Default {
                        }
                        frame 1 {
                        }
                      }
                    }
                    frame 1 {
                      n269 = call <vilib>:"Std Deviation and Variance.vi"("X"=w394) -> ("mean"=w393:dbl, "standard deviation"=w392:dbl)  [unwired: 1 in, 1 out]
                    }
                    frame 2 {
                      n270 = call-poly <vilib>:"RMS.vi"("X"=w397) -> ("rms value"=w395:dbl)  [unwired: 1 out]
                      n271 = case shown="0, Default" w396 {
                        tunnel: [w399 w401] -> w398
                        tunnel: w397 -> [w400 w405]
                        tunnel: w395 -> [_ w404]
                        frame 0, Default {
                          n272 = call <vilib>:"Std Deviation and Variance.vi"("X"=w400) -> ("standard deviation"=w399:dbl)  [unwired: 1 in, 2 out]
                        }
                        frame 1 {
                          n273 = for {
                            tunnel: w405 -> [w413] mode=indexing
                            tunnel: w404 -> [w414]
                            shift-right: [w409] -> w403
                            shift-left: 0.0 -> [w408]
                            n274 = Square(x=w414) -> (x^2=w412:dbl)
                            n275 = Square(x=w413) -> (x^2=w411:dbl)
                            n276 = Subtract(x=w412, y=w411) -> (x-y=w410:dbl)
                            n277 = Square(x=w410) -> (x^2=w407:dbl)
                            n278 = Add(x=w408, y=w407) -> (x+y=w409:dbl)
                          }
                          n279 = Square Root(x=w403) -> (sqrt(x)=w402:dbl)
                          n280 = Square Root(x=w402) -> (sqrt(x)=w401:dbl)
                        }
                      }
                    }
                  }
                }
              }
            }
            n281 = for {
              tunnel: w340 -> [w421] mode=indexing
              tunnel: [w422] -> w339 mode=indexing
              tunnel: w334 -> [w420] mode=indexing
              tunnel: w329 -> [w419] mode=indexing
              n282 = Bundle("x"=w420, "rms value"=w421, "rms value"=w419) -> (w422:T7)  [unwired: 1 out]
            }
            n283 = for {
              tunnel: w333 -> [w417] mode=indexing
              tunnel: [w418] -> w335 mode=indexing
              tunnel: w334 -> [w416] mode=indexing
              tunnel: w328 -> [w415] mode=indexing
              n284 = Bundle("x"=w416, "standard deviation"=w417, "standard deviation"=w415) -> (w418:T8)  [unwired: 1 out]
            }
            n285 = Sort 1D Array(array=w339) -> (sorted array=w326:T9)
            n286 = Sort 1D Array(array=w335) -> (sorted array=w325:T10)
          }
        }
        n287 = Bundle By Name(cluster=w62, "Curve"=w71, "single val"=w61, "Name"=w77, "Step No."=w72) -> (w78:T2)
        n288 = Bundle By Name(cluster=w62, "Curve"=w70, "single val"=w61, "Name"=w76, "Step No."=w72) -> (w75:T2)
      }
    }
    n289 = call "CRYConvertWorkinValue.vi"("Work in"=w19, "In"=w28, "Type"=w31) -> ("Out"=w27:T2)  [unwired: 8 in]
    n290 = call "CRYConvertWorkinValue.vi"("Work in"=w19, "In"=w32, "Type"=w31) -> ("Out"=w30:T2)  [unwired: 8 in]
  }
  "Mean Out" <- w14
  "Absolute StanDev Out" <- w13
  "Out F" <- FALSE ("Out F")
